vi "create image core.vi"(10 "Project Path":path, 11 "Destination":path) -> (0 "error out":errorcluster)   [LabVIEW 2014]
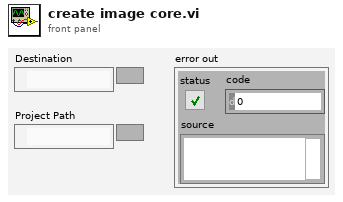
[diagram p1: front panel]
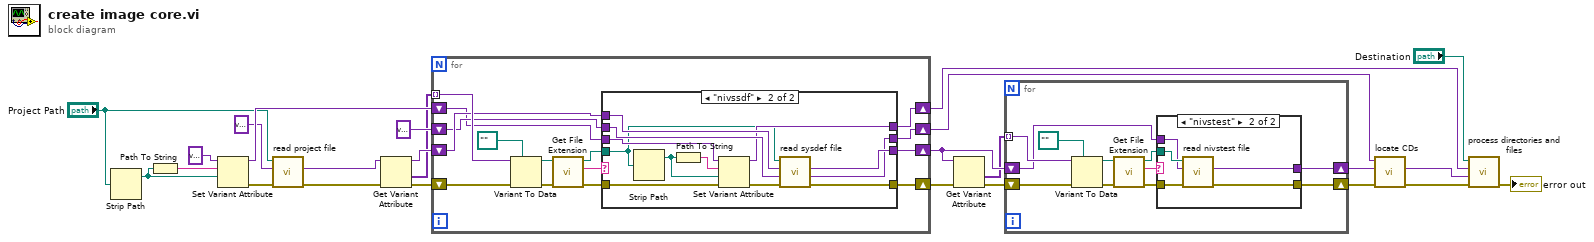
[diagram p0: block diagram]
diagram:
  n1 = Strip Path(path="Project Path") -> (stripped path=w16:path)  [unwired: 1 out]
  n2 = Path To String(path=w16) -> (string=w15:string)
  n3 = Set Variant Attribute(Variant=variant ("variant"), name=w15, value=w16) -> (Variant out=w17:variant, error out=w14:errorcluster)  [unwired: 1 in, 1 out]
  n4 = call "read project file.vi"("error in (no error)"=w14, "lookup in"=variant, "Path"="Project Path") -> ("error out"=w1:errorcluster, "lookup out"=w4:variant)  [unwired: 7 in]
  n5 = Get Variant Attribute(Variant=w4, error in=w1) -> (duplicate Variant=w6:variant, values=w5:variant[], error out=w3:errorcluster)  [unwired: 2 in, 1 out]
  n6 = for {
    shift-right: [w37] -> w8
    shift-left: w3 -> [w36]
    tunnel: w5 -> [w34] mode=indexing
    shift-right: [w30] -> w11
    shift-left: w6 -> [w31]
    shift-right: [w29] -> w20
    shift-left: variant ("CD list out") -> [w28]
    shift-right: [w26] -> w23
    shift-left: w17 -> [w27]
    n7 = Variant To Data(error in=w36, type=path "", Variant=w34) -> (data=w33:path, error out=w35:errorcluster)
    n8 = call <vilib>:"Get File Extension.vi"("error in (no error)"=w35, "file"=w33) -> ("error out"=w38:errorcluster, "lowercase file extension"=w40:string, "dup file"=w39:path)  [unwired: 6 in, 1 out]
    n9 = case shown="\"nivssdf\"" w40 {
      tunnel: w39 -> [_ w47]
      tunnel: w38 -> [w44 w46]
      tunnel: [w44 w56] -> w37
      tunnel: [w43 w55] -> w30
      tunnel: w31 -> [w43 w54]
      tunnel: [w42 w53] -> w29
      tunnel: w28 -> [w42 w52]
      tunnel: w27 -> [w41 w51]
      tunnel: [w41 w50] -> w26
      frame Default {
      }
      frame "nivssdf" {
        n10 = Strip Path(path=w47) -> (stripped path=w48:path)  [unwired: 1 out]
        n11 = Path To String(path=w48) -> (string=w49:string)
        n12 = Set Variant Attribute(Variant=w51, name=w49, value=w48, error in=w46) -> (Variant out=w50:variant, error out=w45:errorcluster)  [unwired: 1 out]
        n13 = call "read sysdef file.vi"("error in (no error)"=w45, "CD list in"=w52, "lookup in"=w54, "Path"=w47) -> ("error out"=w56:errorcluster, "CD list out"=w53:variant, "lookup out"=w55:variant)  [unwired: 5 in]
      }
    }
  }
  n14 = Get Variant Attribute(Variant=w11, error in=w8) -> (values=w10:variant[], error out=w9:errorcluster)  [unwired: 2 in, 2 out]
  n15 = for {
    shift-right: [w64] -> w18
    shift-left: w9 -> [w63]
    tunnel: w10 -> [w61] mode=indexing
    shift-right: [w57] -> w19
    shift-left: w11 -> [w58]
    n16 = Variant To Data(error in=w63, type=path "", Variant=w61) -> (data=w60:path, error out=w62:errorcluster)
    n17 = call <vilib>:"Get File Extension.vi"("error in (no error)"=w62, "file"=w60) -> ("error out"=w65:errorcluster, "lowercase file extension"=w67:string, "dup file"=w66:path)  [unwired: 6 in, 1 out]
    n18 = case shown="\"nivstest\"" w67 {
      tunnel: w66 -> [_ w73]
      tunnel: w65 -> [w69 w74]
      tunnel: [w69 w70] -> w64
      tunnel: [w68 w71] -> w57
      tunnel: w58 -> [w68 w72]
      frame Default {
      }
      frame "nivstest" {
        n19 = call "read nivstest file.vi"("error in (no error)"=w74, "lookup in"=w72, "Path"=w73) -> ("error out"=w70:errorcluster, "lookup out"=w71:variant)  [unwired: 7 in]
      }
    }
  }
  n20 = call "locate CDs.vi"("error in (no error)"=w18, "include files in"=w19, "cds"=w20) -> ("error out"=w21:errorcluster, "include files out"=w22:variant)  [unwired: 7 in]
  n21 = call "process directories and files.vi"("error in"=w21, "include files in"=w22, "include directories"=w23, "Destination directory"="Destination") -> ("error out"=→"error out":errorcluster)  [unwired: 7 in]
